vi "Get Pin Status.vi"(8 "error in (no error)":errorcluster, 9 "Pin":string, 10 "Puerto":string, 11 "UI Actor in":refnum<class "UI Actor.lvclass">) -> (0 "error out":errorcluster, 3 "UI Actor out":refnum<class "UI Actor.lvclass">)   [LabVIEW 2020, in "UI Actor.lvlib" / "UI Actor.lvclass"]
uses:
  UI Actor.lvclass
  UI Actor.lvclass/UI Actor.ctl
  Abstract/Serial Device/Serial Device.lvclass
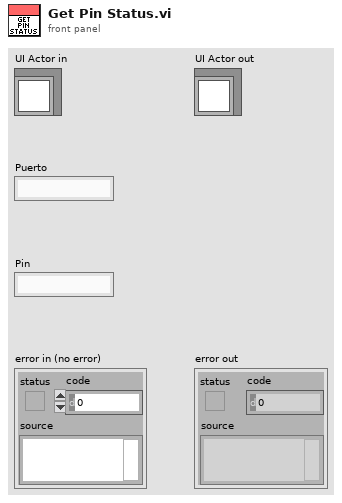
[diagram p1: front panel]
types:
  T1 = typedef "Control 1.ctl" = string
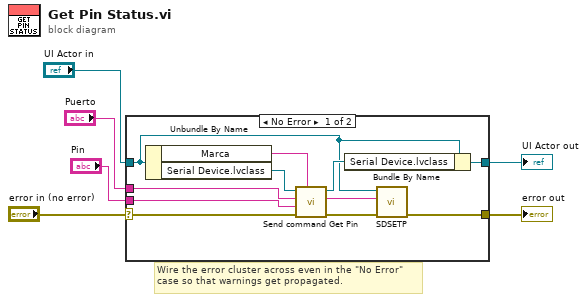
[diagram p0: block diagram]
diagram:
  # "Wire the error cluster across even in the \"No Error\"\ncase so that warnings get propagated."
  n1 = case shown="No Error" "error in (no error)" {
    selector: "error in (no error)" -> [w15 w19]
    tunnel: [w9 w19] -> w5
    tunnel: [w14 w18] -> w3
    tunnel: "UI Actor in" -> [w8 w18]
    tunnel: "Puerto" -> [w12 _]
    tunnel: "Pin" -> [w11 _]
    frame No Error {
      n2 = Unbundle By Name(w8) -> ("Marca"=w16:T1, "Serial Device.lvclass"=w17:refnum<class "Serial Device.lvclass">)
      n3 = call-dynamic "Send command Get Pin.vi"("Marca"=w16, "error in (no error)"=w15, "Pin"=w11, "Puerto"=w12, "Serial Device in"=w17) -> ("error out"=w10:errorcluster, "Expected response"=w7:string, "Serial Device out"=w13:refnum<class "Serial Device.lvclass">)  [unwired: 3 in, 1 out]
      n4 = Bundle By Name(cluster=w8, "Serial Device.lvclass"=w13) -> (w14:refnum<class "UI Actor.lvclass">)
      n5 = call "SDSETP.vi"("error in (no error)"=w10, "Expected response"=w7, "UI Actor in"=w8) -> ("error out"=w9:errorcluster)  [unwired: 8 in]
    }
    frame Error {
    }
  }
  "error out" <- w5
  "UI Actor out" <- w3
